vi "Get DataArray.vi"   [LabVIEW 2016, in "DataGrid.lvlib" / "DataGridView.lvclass"]
uses:
  <userlib>/LabVIEWdotNetDataGrid/source/DataGridView/DataGridView.lvclass
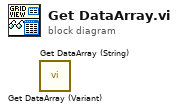
[diagram p0: block diagram]
diagram:
  n1 = call <userlib>:"Get DataArray (String).vi"() -> ()  [unwired: 9 in, 3 out]
  n2 = call <userlib>:"Get DataArray (Variant).vi"() -> ()  [unwired: 9 in, 3 out]
